vi "DirettoreStart.vi"(11 "FPGAReference":refnum<k20>) -> (0 "ErrorOut":errorcluster)   [LabVIEW 2012]
uses:
  <vilib>/FPGAPlugInAG/Dynamic/niLvFpga_Reset_Dynamic.vi
  <vilib>/FPGAPlugInAG/Dynamic/niLvFpga_Run_Dynamic.vi
  <vilib>/rvi/interface/nirviMethod/nirviMethod.xnode
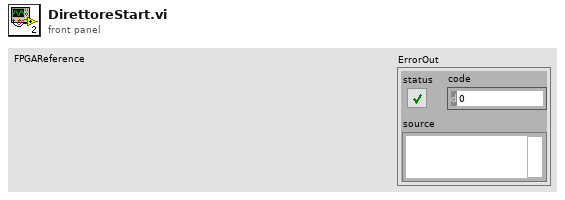
[diagram p1: front panel]
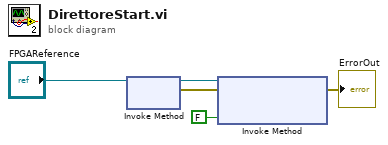
[diagram p0: block diagram]
diagram:
  n1 = xnode "Invoke Method"("FPGA VI Reference In"="FPGAReference") -> ("FPGA VI Reference Out"=w2:refnum<k20>, "error out"=w1:errorcluster)  [unwired: 1 in]
  n2 = xnode "Invoke Method"("FPGA VI Reference In"=w2, "error in"=w1, "Wait Until Done (F)"=FALSE) -> ("error out"=→"ErrorOut":errorcluster)  [unwired: 1 out]
